vi "ArmPathLength.vi"(0 "Angles":dbl[](array[numeric]), 3 "Radii":dbl[](array[numeric])) -> (1 "Path Length":dbl, 2 "Angles Out":dbl[](array[numeric]), 4 "IndexedPathLength":dbl[](array[numeric]), 5 "Radii Out":dbl[](array[numeric]))   [LabVIEW 2017]
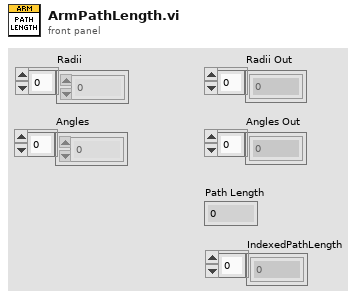
[diagram p1: front panel]
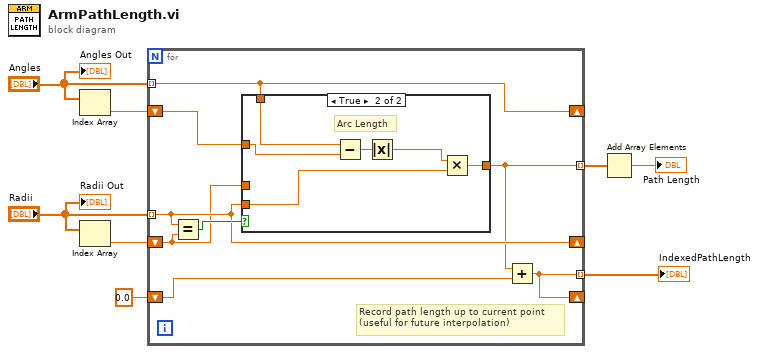
[diagram p0: block diagram]
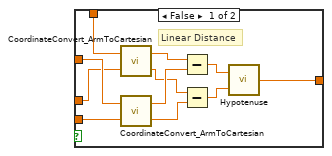
[diagram p2: hidden frame]
diagram:
  n1 = Index Array(array="Angles") -> (element=w7:dbl)  [unwired: 1 in]
  n2 = Index Array(array="Radii") -> (element=w6:dbl)  [unwired: 1 in]
  n3 = for {
    tunnel: "Angles" -> [w15] mode=indexing
    tunnel: "Radii" -> [w13] mode=indexing
    shift-right: [w13] -> _
    shift-left: w6 -> [w12]
    shift-right: [w15] -> _
    shift-left: w7 -> [w14]
    tunnel: [w10] -> w5 mode=indexing
    shift-right: [w11] -> _
    shift-left: 0.0 -> [w9]
    tunnel: [w11] -> w1 mode=indexing
    # "Record path length up to current point\n(useful for future interpolation)"
    n4 = Equal?(x=w13, y=w12) -> (x = y?=w16:bool)
    n5 = case shown="True" w16 {
      tunnel: w15 -> [w20 w31]
      tunnel: w12 -> [w18 _]
      tunnel: w13 -> [w17 w28]
      tunnel: [w21 w32] -> w10
      tunnel: w14 -> [w19 w30]
      frame False {
        # "Linear Distance"
        n6 = call "CoordinateConvert_ArmToCartesian.vi"("Radius (in)"=w18, "Angle (rad)"=w20) -> ("Y (in)"=w25:dbl, "X (in)"=w27:dbl)
        n7 = call "CoordinateConvert_ArmToCartesian.vi"("Radius (in)"=w17, "Angle (rad)"=w19) -> ("Y (in)"=w24:dbl, "X (in)"=w26:dbl)
        n8 = Subtract(x=w27, y=w26) -> (x-y=w23:dbl)
        n9 = Subtract(x=w25, y=w24) -> (x-y=w22:dbl)
        n10 = call "Hypotenuse.vi"("Y"=w22, "X"=w23) -> ("Hypotenuse"=w21:dbl)
      }
      frame True {
        # "Arc Length"
        n11 = Subtract(x=w31, y=w30) -> (x-y=w33:dbl)
        n12 = Absolute Value(x=w33) -> (abs(x)=w29:dbl)
        n13 = Multiply(x=w29, y=w28) -> (x*y=w32:dbl)
      }
    }
    n14 = Add(x=w10, y=w9) -> (x+y=w11:dbl)
  }
  "IndexedPathLength" <- w1
  n15 = Add Array Elements(numeric array=w5) -> (sum=→"Path Length":dbl)
  "Radii Out" <- "Radii"
  "Angles Out" <- "Angles"
